vi "Configure Function.vi"(8 "error in (no error)":errorcluster, 10 "Function":u16(ring) items=["CURRent", "RESistance", "VOLTage", "POWer"], 11 "VISA resource name":refnum<visa-resource-name>) -> (0 "error out":errorcluster, 3 "VISA resource name out":refnum<visa-resource-name>)   [LabVIEW 2015, in "IT8900A-E.lvlib"]
doc: "This writes the equivalent command to select load adjustment mode.\nCURRent constant CURRent mode\nhold constant hold mode\nVOLTage constant VOLTage mode\nPOWer constant POWer mode"
uses:
  <instrlib>/IT8900/IT8900A-E.lvlib
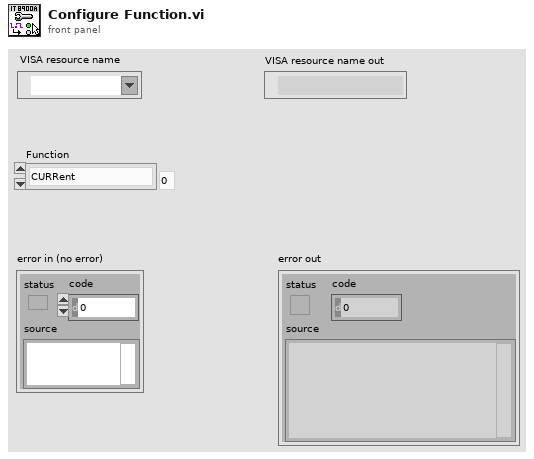
[diagram p1: front panel]
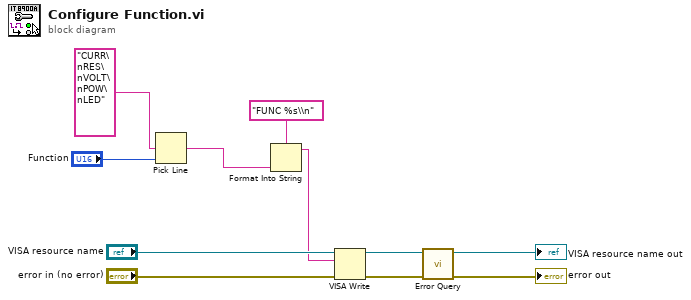
[diagram p0: block diagram]
diagram:
  n1 = Pick Line(multi-line string="CURR\nRES\nVOLT\nPOW\nLED", line index="Function") -> (output string=w3:string)  [unwired: 1 in]
  n2 = Format Into String(format string="FUNC %s\\n", w3) -> (resulting string=w5:string)  [unwired: 2 in, 1 out]
  n3 = VISA Write(VISA resource name="VISA resource name", write buffer=w5, error in (no error)="error in (no error)") -> (VISA resource name out=w8:refnum<visa-resource-name>, error out=w10:errorcluster)  [unwired: 1 out]
  n4 = call <instrlib>:"Error Query.vi"("error in (no error)"=w10, "VISA resource name"=w8) -> ("error out"=→"error out":errorcluster, "VISA resource name out"=→"VISA resource name out":refnum<visa-resource-name>)  [unwired: 6 in, 2 out]
